vi "listener.vi"(10 "parameters":T1, 11 "websocket standalone server in":refnum<class "websocket standalone server.lvclass">) -> ()   [LabVIEW 2016, in "websocket standalone server.lvclass"]
uses:
  websocket standalone server.lvclass
  websocket connection parameters.ctl
  websocket standalone server.lvclass/websocket standalone server.ctl
  websocket data packet.ctl
  websocket message type.ctl
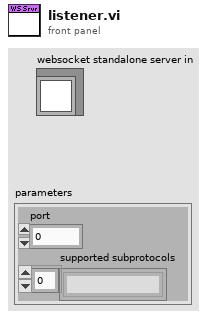
[diagram p1: front panel]
types:
  T1 = typedef "websocket standalone server.lvclass/websocket connection parameters.ctl" = cluster{"port":u16, "supported subprotocols":string[]}
  T2 = typedef "websocket standalone server.lvclass/websocket data packet.ctl" = cluster{"message type":T3, "data":string}
  T3 = typedef "websocket standalone server.lvclass/websocket message type.ctl" = enum16{"UTF8 data", "binary data", "close", "ping", "pong"}
  T4 = typedef "websocket standalone server.lvclass/websocket listener message.ctl" = enum16{"exit", "block socket", "unblock socket"}
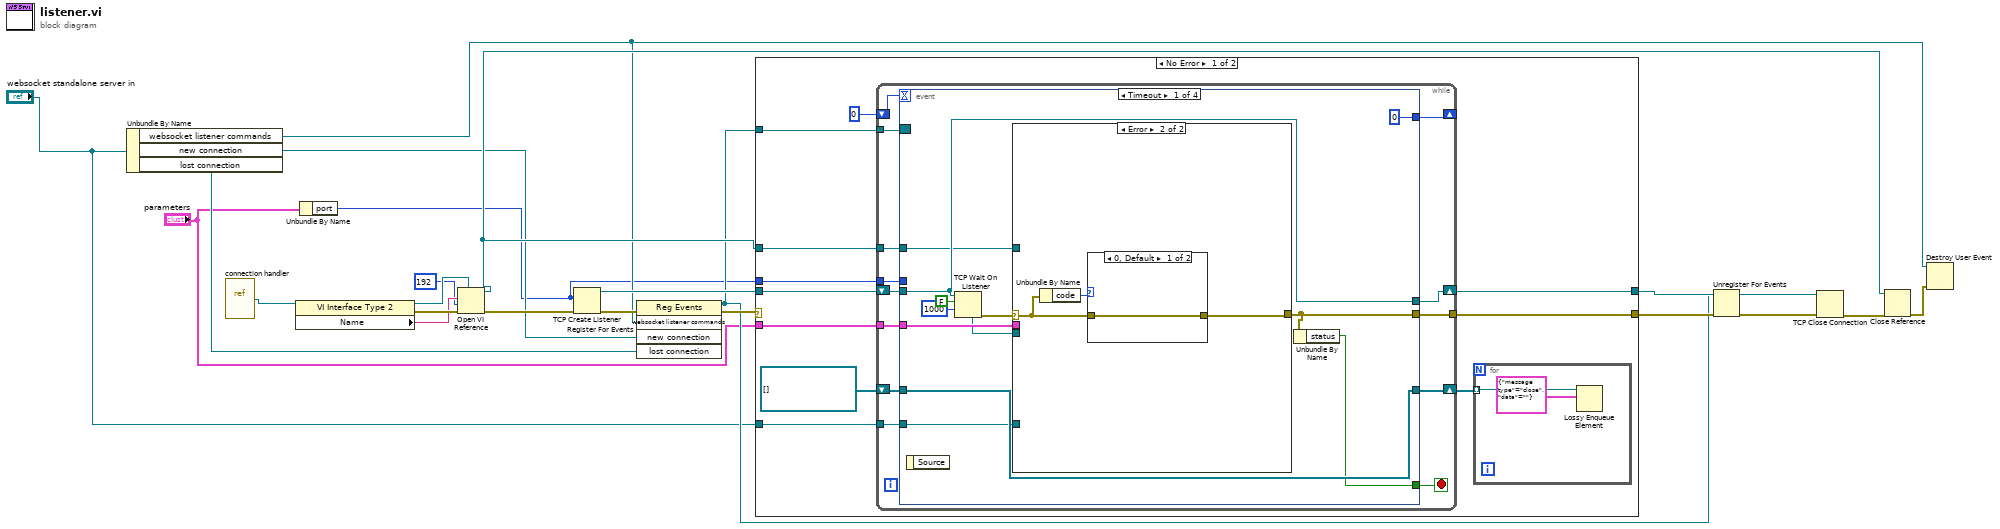
[diagram p0: block diagram]
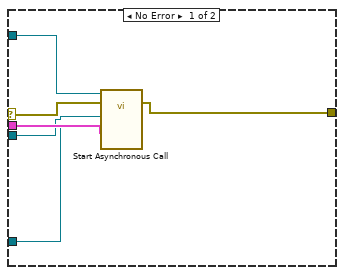
[diagram p2: hidden frame]
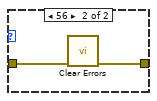
[diagram p3: hidden frame]
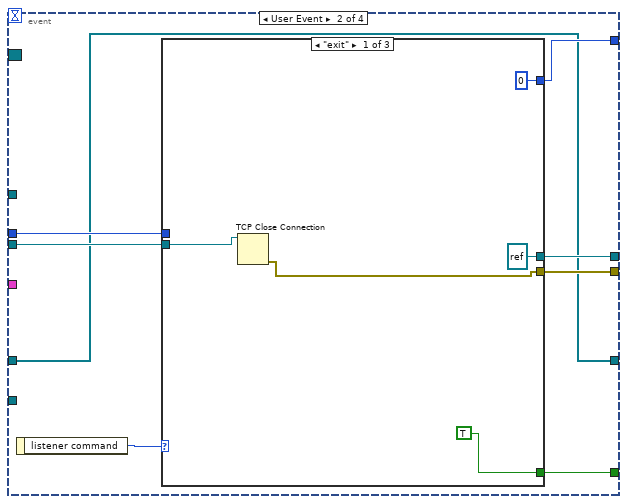
[diagram p4: hidden frame]
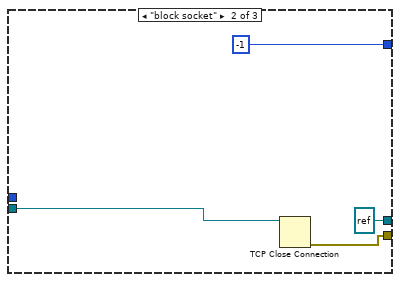
[diagram p5: hidden frame]
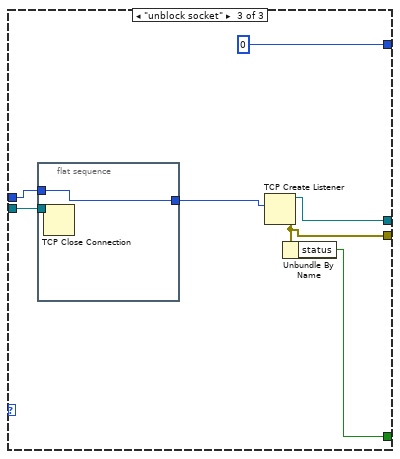
[diagram p6: hidden frame]
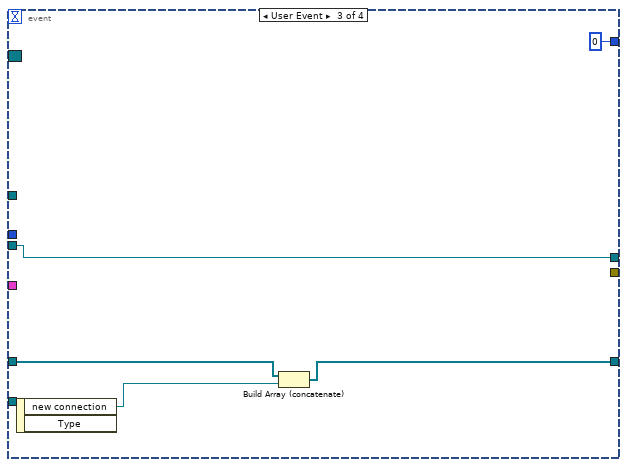
[diagram p7: hidden frame]
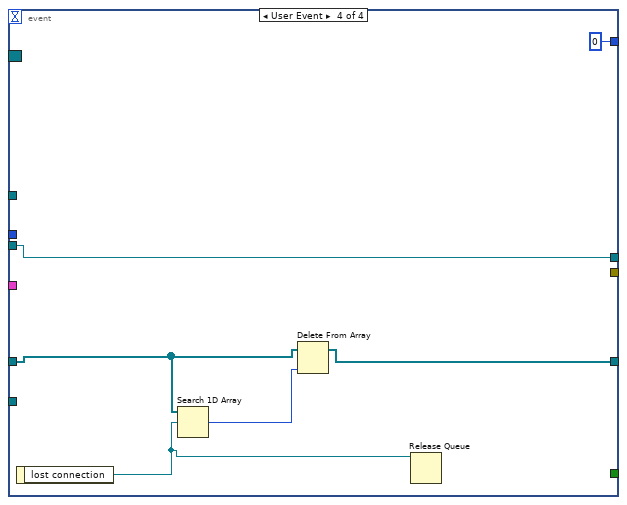
[diagram p8: hidden frame]
diagram:
  n1 = Unbundle By Name("websocket standalone server in") -> ("websocket listener commands"=w7:refnum<user-event>, "new connection"=w6:refnum<user-event>, "lost connection"=w5:refnum<user-event>)
  n2 = vi-ref "connection handler.vi"() -> (w22:refnum<vi>)
  n3 = property class="VI Interface Type 2"(reference=w22) -> (reference out=w19:refnum<vi>, error out=w21:errorcluster, "Name"=w20:string)  [unwired: 1 in]
  n4 = Unbundle By Name("parameters") -> ("port"=w3:u16)
  n5 = Open VI Reference(type specifier VI Refnum (for type only)=w19, vi path=w20, options=192, error in (no error)=w21) -> (vi reference=w11:refnum<vi>, error out=w17:errorcluster)  [unwired: 2 in]
  n6 = TCP Create Listener(8:w17, 10:w3) -> (0:w16:errorcluster, 3:w14:refnum<k5>)  [unwired: 3 in, 1 out]
  n7 = register-events(error in=w16, w7, w6, w5) -> (reference out=w4:refnum<event-registration>, error out=w9:errorcluster)  [unwired: 1 in]
  n8 = case shown="No Error" w9 {
    selector: w9 -> [_ w110]
    tunnel: [w27 w111] -> w15
    tunnel: w14 -> [w33 w111]
    tunnel: [w25 w110] -> w13
    tunnel: w11 -> [w32 _]
    tunnel: w4 -> [w30 _]
    tunnel: w3 -> [w26 _]
    tunnel: "parameters" -> [w24 _]
    tunnel: "websocket standalone server in" -> [w23 _]
    frame No Error {
      n9 = while {
        shift-right: [w43] -> w27
        shift-left: w33 -> [w48]
        tunnel: w32 -> [w47]
        shift-right: [w45] -> _
        shift-left: 0 -> [w46]
        tunnel: w30 -> [w44]
        shift-right: [w38] -> w28
        shift-left: refnum<queue>[] [] -> [w41]
        tunnel: w26 -> [w40]
        tunnel: [w39] -> w25
        tunnel: w24 -> [w37]
        tunnel: w23 -> [w36]
        stop <- w42 stop-if-true
        n10 = event shown="[0] Timeout" {
          selector: w44 -> [_ _ _ _]
          dyn-events: _ -> [_ _ _ _]
          timeout: w46 -> [_ _ _ _]
          tunnel: w48 -> [w60 w78 w103 w109]
          tunnel: w47 -> [w57 _ _ _]
          tunnel: [0 w77 0 0] -> w45
          tunnel: [w60 w79 w103 w109] -> w43
          tunnel: [w53 w76 _ _] -> w42
          tunnel: w41 -> [w55 w73 w102 w107]
          tunnel: w40 -> [_ w75 _ _]
          tunnel: [w54 w74 _ _] -> w39
          tunnel: [w55 w73 w100 w108] -> w38
          tunnel: w37 -> [w52 _ _ _]
          tunnel: w36 -> [w51 _ _ _]
          event Timeout {
            n11 = event-data() -> ()  [unwired: 1 in, 1 out]
            n12 = TCP Wait On Listener(9:1000 ("timeout ms (wait forever: -1)"), 10:FALSE ("resolve remote address (T)"), 11:w60) -> (0:w58:errorcluster, 4:w50:refnum<k5>)  [unwired: 1 in, 3 out]
            n13 = case shown="Error" w58 {
              selector: w58 -> [w66 w67]
              tunnel: w57 -> [w65 _]
              tunnel: [w64 w69] -> w54
              tunnel: w52 -> [w63 _]
              tunnel: w51 -> [w62 _]
              tunnel: w50 -> [w61 _]
              frame No Error {
                n14 = call-by-ref "Start Asynchronous Call"(reference=w65, error in=w66, "parameters"=w63, "websocket standalone server in"=w62, "connection ID"=w61) -> (error out=w64:errorcluster)  [unwired: 9 in, 1 out]
              }
              frame Error {
                n15 = Unbundle By Name(w67) -> ("code"=w68:i32)
                n16 = case shown="0, Default" w68 {
                  tunnel: w67 -> [w70 w72]
                  tunnel: [w70 w71] -> w69
                  frame 0, Default {
                  }
                  frame 56 {
                    n17 = call <vilib>:"Clear Errors.vi"("error in (no error)"=w72) -> ("error out"=w71:errorcluster)  [unwired: 5 in, 1 out]
                  }
                }
              }
            }
            n18 = Unbundle By Name(w54) -> ("status"=w53:bool)
          }
          event User Event {
            n19 = event-data() -> ("listener command"=w80:T4)  [unwired: 1 in]
            n20 = case shown="\"exit\"" w80 {
              tunnel: [refnum<k5> refnum ("listener ID") refnum<k5> refnum ("listener ID") w92] -> w79
              tunnel: w78 -> [w83 w89 w96]
              tunnel: [0 -1 0] -> w77
              tunnel: [TRUE _ w91] -> w76
              tunnel: w75 -> [_ _ w94]
              tunnel: [w81 w86 w90] -> w74
              frame "exit" {
                n21 = TCP Close Connection(connection ID=w83) -> (error out=w81:errorcluster)  [unwired: 2 in, 1 out]
              }
              frame "block socket" {
                n22 = TCP Close Connection(connection ID=w89) -> (error out=w86:errorcluster)  [unwired: 2 in, 1 out]
              }
              frame "unblock socket" {
                n23 = flat-sequence {
                  tunnel: w96 -> [w98]
                  tunnel: w94 -> [w97]
                  tunnel: [w97] -> w93
                  frame #0 {
                    n24 = TCP Close Connection(connection ID=w98) -> ()  [unwired: 2 in, 2 out]
                  }
                }
                n25 = TCP Create Listener(10:w93) -> (0:w90:errorcluster, 3:w92:refnum<k5>)  [unwired: 4 in, 1 out]
                n26 = Unbundle By Name(w90) -> ("status"=w91:bool)
              }
            }
          }
          event User Event {
            n27 = event-data() -> ("new connection"=w101:refnum<queue>)  [unwired: 1 in, 1 out]
            n28 = Build Array (concatenate)(w102, w101) -> (w100:refnum<queue>[])
          }
          event User Event {
            n29 = event-data() -> ("lost connection"=w105:refnum<queue>)  [unwired: 1 in]
            n30 = Search 1D Array(1D array=w107, element=w105) -> (index of element=w106:i32)  [unwired: 1 in]
            n31 = Delete From Array(array=w107, index=w106) -> (array with subset deleted=w108:refnum<queue>[])  [unwired: 1 in, 1 out]
            n32 = Release Queue(queue=w105) -> ()  [unwired: 2 in, 3 out]
          }
        }
      }
      n33 = for {
        tunnel: w28 -> [w35] mode=indexing
        n34 = Lossy Enqueue Element(queue=w35, element=T2 {"message type"=enum."close", "data"=""}) -> ()  [unwired: 1 in, 4 out]
      }
    }
    frame Error {
    }
  }
  n35 = Unregister For Events(event registration refnum=w4, error in=w13) -> (error out=w8:errorcluster)
  n36 = TCP Close Connection(connection ID=w15, error in (no error)=w8) -> (error out=w12:errorcluster)  [unwired: 1 in, 1 out]
  n37 = Close Reference(reference=w11, error in (no error)=w12) -> (error out=w10:errorcluster)
  n38 = Destroy User Event(user event=w7, error in=w10) -> ()  [unwired: 1 out]
